vi "HF2LI_Messgerät.vi"(11 "refnum 2":refnum<file>) -> ()   [LabVIEW 2019]
uses:
  Global/Global Variables/Data_Display_global.vi
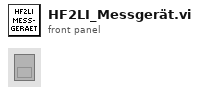
[diagram p1: front panel]
types:
  T1 = typedef "HF2LI.ctl" = cluster{"X 1 (Vrms)":dbl, "Y 1 (Vrms)":dbl, "A 1 (Vpk)":dbl, "A 2 (Vpk)":dbl, "Output 1":bool, "Output 2":bool, "f 1 (Hz)":dbl, "f 2 (Hz)":dbl, "X 2 (Vrms)":dbl, "Y 2 (Vrms)":dbl, "Output 1 Add":bool, "Output 2 Add":bool, "Input Min %":dbl, "Input Max %":dbl}
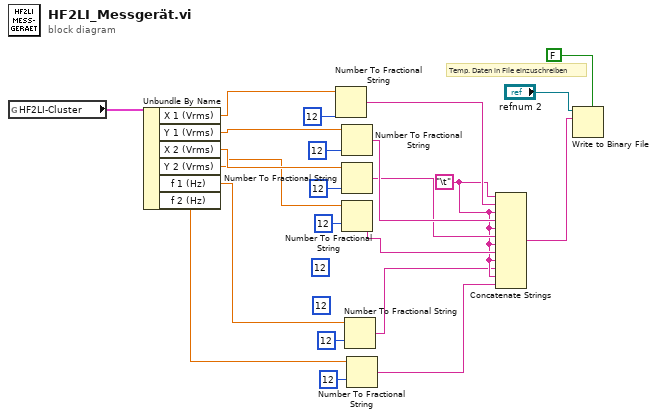
[diagram p0: block diagram]
diagram:
  w6 = "\t"
  (unwired) i16 12 ("precision (6)")
  (unwired) i16 12 ("precision (6)")
  # "Temp. Daten in File einzuschreiben"
  n1 = global read "Data_Display_global.vi" "HF2LI-Cluster"() -> (w23:T1)
  n2 = Unbundle By Name(w23) -> ("X 1 (Vrms)"=w18:dbl, "Y 1 (Vrms)"=w17:dbl, "X 2 (Vrms)"=w14:dbl, "Y 2 (Vrms)"=w13:dbl, "f 1 (Hz)"=w12:dbl, "f 2 (Hz)"=w11:dbl)
  n3 = Number To Fractional String(number=w18, precision (6)=i16 12) -> (F-format string=w10:string)  [unwired: 2 in]
  n4 = Number To Fractional String(number=w17, precision (6)=i16 12) -> (F-format string=w9:string)  [unwired: 2 in]
  n5 = Number To Fractional String(number=w14, precision (6)=i16 12) -> (F-format string=w8:string)  [unwired: 2 in]
  n6 = Number To Fractional String(number=w13, precision (6)=i16 12) -> (F-format string=w7:string)  [unwired: 2 in]
  n7 = Number To Fractional String(number=w12, precision (6)=i16 12) -> (F-format string=w2:string)  [unwired: 2 in]
  n8 = Number To Fractional String(number=w11, precision (6)=i16 12) -> (F-format string=w1:string)  [unwired: 2 in]
  n9 = Concatenate Strings(w6, w10, w6, w9, w6, w8, w6, w7, w6, w2, w6, w1) -> (w3:string)
  n10 = Write to Binary File ("Write File")(file (use dialog)="refnum 2", data=w3, 5:FALSE ("prepend array or string size? (T)")) -> ()  [unwired: 3 in, 3 out]
